vi "get channel index from channel selector values.vi"(9 "channelSelection":T1 {"oilP" items=["time", "gearbox", "Recirculation temp", "volute exit surface", "oil tank", "Inlet average", "Outlet average", "V-cone", "inlet pressure", "outlet pressure", "Motor speed", "V-cone DP", "Motor power", "Accelerometer", "Hotwire", "oil pressure", "butterfly valve position", "Legacy speed", "new Vcone", "ambient pressure", "ambient temperature"]; "ballControl" items=["ball valve drive", "Motor Speed", "", "butterfly valve drive"]; "butterflyControl" items=["ball valve drive", "Motor Speed", "", "butterfly valve drive"]; "speedControl" items=["ball valve drive", "Motor Speed", "", "butterfly valve drive"]; "speedFeedback" items=["time", "gearbox", "Recirculation temp", "volute exit surface", "oil tank", "Inlet average", "Outlet average", "V-cone", "inlet pressure", "outlet pressure", "Motor speed", "V-cone DP", "Motor power", "Accelerometer", "Hotwire", "oil pressure", "butterfly valve position", "Legacy speed", "new Vcone", "ambient pressure", "ambient temperature"]; "ballValue" items=["time", "gearbox", "Recirculation temp", "volute exit surface", "oil tank", "Inlet average", "Outlet average", "V-cone", "inlet pressure", "outlet pressure", "Motor speed", "V-cone DP", "Motor power", "Accelerometer", "Hotwire", "oil pressure", "butterfly valve position", "Legacy speed", "new Vcone", "ambient pressure", "ambient temperature"]; "butterflyValue" items=["time", "gearbox", "Recirculation temp", "volute exit surface", "oil tank", "Inlet average", "Outlet average", "V-cone", "inlet pressure", "outlet pressure", "Motor speed", "V-cone DP", "Motor power", "Accelerometer", "Hotwire", "oil pressure", "butterfly valve position", "Legacy speed", "new Vcone", "ambient pressure", "ambient temperature"]; "masflow" items=["time", "gearbox", "Recirculation temp", "volute exit surface", "oil tank", "Inlet average", "Outlet average", "V-cone", "inlet pressure", "outlet pressure", "Motor speed", "V-cone DP", "Motor power", "Accelerometer", "Hotwire", "oil pressure", "butterfly valve position", "Legacy speed", "new Vcone", "ambient pressure", "ambient temperature"]; "pressureRatio" items=["time", "gearbox", "Recirculation temp", "volute exit surface", "oil tank", "Inlet average", "Outlet average", "V-cone", "inlet pressure", "outlet pressure", "Motor speed", "V-cone DP", "Motor power", "Accelerometer", "Hotwire", "oil pressure", "butterfly valve position", "Legacy speed", "new Vcone", "ambient pressure", "ambient temperature"]}, 11 "controls in":T2 {"allValues"."safetyLimits"."channelLimits"."channelID" items=["time", "gearbox", "compressor bearing", "shaft bearing", "oil outlet", "inlet 1", "inlet 2", "outlet 1", "outlet 2", "inlet pressure", "outlet pressure", "plenum pressure", "Motor speed", "new V-cone DP", "Motor power", "Accelerometer", "Hotwire 1", "oil pressure", "butterfly valve position", "ball valve position", "Legacy speed", "Torque speed", "pulsator encoder", "v-cone upstream 1", "v-cone upstream 2"]}) -> (3 "controls out":T2 {"allValues"."safetyLimits"."channelLimits"."channelID" items=["time", "gearbox", "compressor bearing", "shaft bearing", "oil outlet", "inlet 1", "inlet 2", "outlet 1", "outlet 2", "inlet pressure", "outlet pressure", "plenum pressure", "Motor speed", "new V-cone DP", "Motor power", "Accelerometer", "Hotwire 1", "oil pressure", "butterfly valve position", "ball valve position", "Legacy speed", "Torque speed", "pulsator encoder", "v-cone upstream 1", "v-cone upstream 2"]})   [LabVIEW 2018]
uses:
  systemConfigUIControls.ctl
  type defs/channelLimitControl.ctl
  type defs/limitActions.ctl
  ICL-LabVIEW_General/data channels/parent class/Data Channel.lvclass
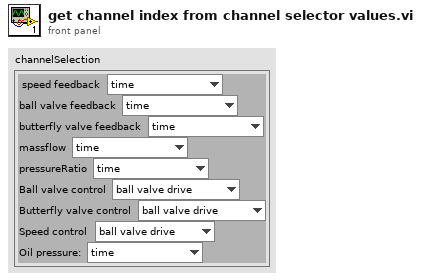
[diagram p1: front panel]
types:
  T1 = cluster{"speedFeedback":u16, "ballValue":u16, "butterflyValue":u16, "masflow":u16, "pressureRatio":u16, "ballControl":u16, "butterflyControl":u16, "speedControl":u16, "oilP":u16}
  T2 = typedef "systemConfigUIControls.ctl" = cluster{"allControls":cluster{"feedbackChannels":cluster{"butterfly":refnum<vi>, "ball":refnum<vi>, "massflow":refnum<vi>, "pressureRatio":refnum<vi>, "airP":refnum<vi>, "water":refnum<vi>, "oilP":refnum<vi>, "speed":refnum<vi>}, "controlChannels":cluster{"butterflyControl":refnum<vi>, "ballControl":refnum<vi>, "speedControl":refnum<vi>}, "channelLimits":refnum<vi>, "pulsatorIP":string}, "allValues":cluster{"feedback":cluster{"butterfly":u16, "ball":u16, "massflow":u16, "pressureRatio":u16, "airP":u16, "water":u16, "oilP":u16, "speed":u16}, "paths":cluster{"channelConfig":path, "systemConfig":path, "incidentLogfile":path, "startFolder":path, "customVI":path}, "RT":cluster{"RTIP":string, "errorReaderName":string, "errorWriterName":string, "errorBufferSize":u16, "commandWriterName":string, "commandReaderName":string, "commandBufferSize":u16, "dataBufferSize":u16, "dataReaderName":string, "dataWriterName":string, "dataBufferLength":u16, "scanivalveIP":string, "scanPeriod":u16}, "controls":cluster{"butterflyControl":u16, "ballControl":u16, "speedControl":u16}, "safetyLimits":cluster{"channelLimits":T3[], "maxSpeed":u32}, "Howden":cluster{"howdenAir":bool, "howden%":dbl}}, "variables":cluster{"feedbackChannelIDs":u16[], "controlChannelIDs":u16[], "channelsArray":refnum<class "Data Channel.lvclass">[]}}
  T3 = typedef "channelLimitControl.ctl" = cluster{"channelID":u16, "Enabled":bool, "warnValue":dbl, "limitValue":dbl, "Invert":bool, "limitAction":T4}
  T4 = typedef "limitActions.ctl" = enum16{"stop", "shutdown", "ignore"}
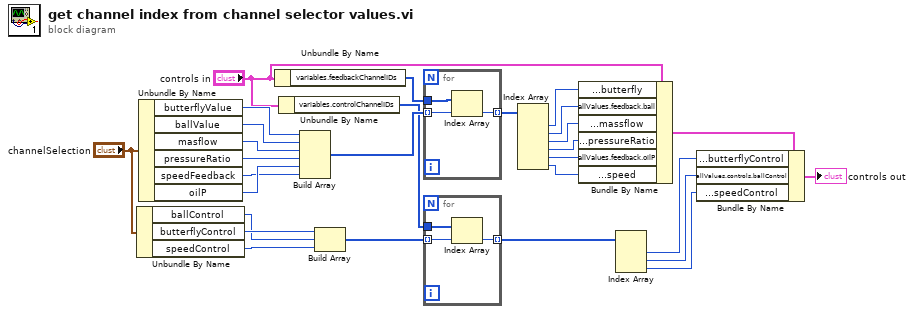
[diagram p0: block diagram]
diagram:
  n1 = Unbundle By Name("channelSelection") -> ("ballControl"=w6:u16, "butterflyControl"=w7:u16, "speedControl"=w10:u16)
  n2 = Unbundle By Name("channelSelection") -> ("butterflyValue"=w28:u16, "ballValue"=w27:u16, "masflow"=w26:u16, "pressureRatio"=w25:u16, "speedFeedback"=w23:u16, "oilP"=w24:u16)
  n3 = Unbundle By Name("controls in") -> ("variables.feedbackChannelIDs"=w11:u16[])
  n4 = Unbundle By Name("controls in") -> ("variables.controlChannelIDs"=w1:u16[])
  n5 = Build Array(w28, w27, w26, w25, w24, w23) -> (w22:u16[])
  n6 = Build Array(w7, w6, w10) -> (w12:u16[])
  n7 = for {
    tunnel: w11 -> [w31]
    tunnel: w22 -> [w30] mode=indexing
    tunnel: [w29] -> w21 mode=indexing
    n8 = Index Array(array=w31, index=w30) -> (element=w29:u16)
  }
  n9 = for {
    tunnel: w1 -> [w34]
    tunnel: w12 -> [w33] mode=indexing
    tunnel: [w32] -> w13 mode=indexing
    n10 = Index Array(array=w34, index=w33) -> (element=w32:u16)
  }
  n11 = Index Array(array=w21) -> (element #1=w20:u16, element #2=w19:u16, element #3=w18:u16, element #4=w17:u16, element #5=w16:u16, element #6=w15:u16)  [unwired: 6 in]
  n12 = Bundle By Name(cluster="controls in", "allValues.feedback.butterfly"=w20, "allValues.feedback.ball"=w19, "allValues.feedback.massflow"=w18, "allValues.feedback.pressureRatio"=w17, "allValues.feedback.oilP"=w16, "allValues.feedback.speed"=w15) -> (w9:T2)
  n13 = Index Array(array=w13) -> (element #1=w5:u16, element #2=w4:u16, element #3=w3:u16)  [unwired: 3 in]
  n14 = Bundle By Name(cluster=w9, "allValues.controls.butterflyControl"=w5, "allValues.controls.ballControl"=w4, "allValues.controls.speedControl"=w3) -> (→"controls out":T2)
